vi "Init DB-Engine.vi"(6 "Database":string, 8 "error in":errorcluster, 9 "Password":string, 10 "User":string, 11 "DB-Engine in":refnum<class "DB-Interface.lvclass">) -> (0 "error out":errorcluster, 3 "DB-Engine out":refnum<class "DB-Interface.lvclass">)   [LabVIEW 2020, in "hse-db.lvlib" / "DB-Interface.lvclass"]
doc: "Initialize the class.\n\n____\nHAMPEL SOFTWARE ENGINEERING v1.4.0 (2023-12-19 09:52)"
uses:
  DB-Interface.lvclass
  DB-Interface.lvclass/DB-Interface.ctl
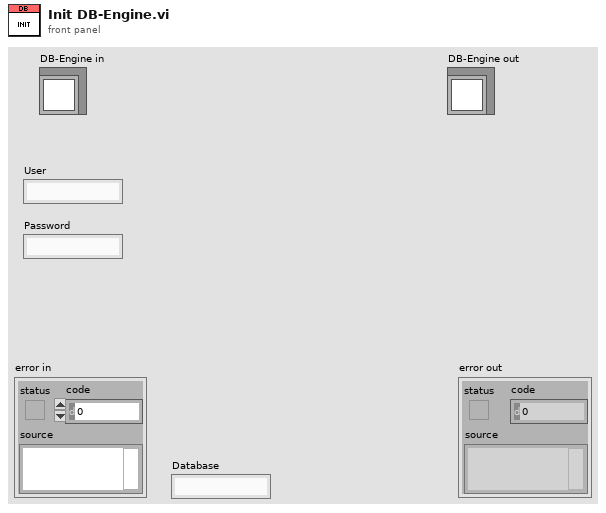
[diagram p1: front panel]
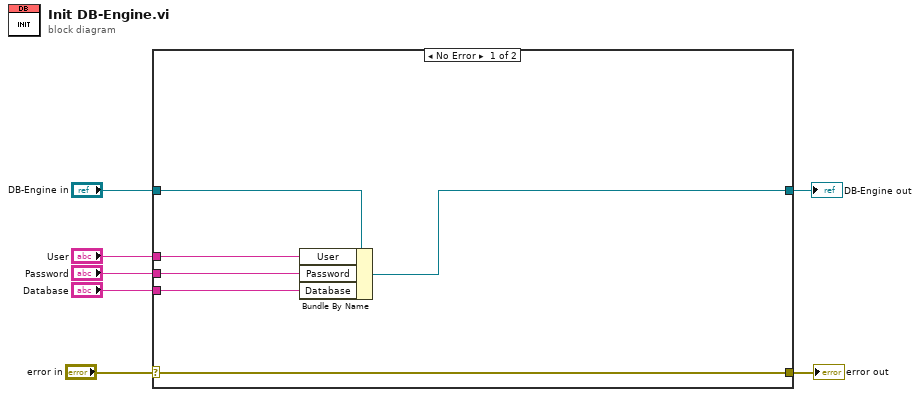
[diagram p0: block diagram]
diagram:
  n1 = case shown="No Error" "error in" {
    selector: "error in" -> [w13 w15]
    tunnel: [w13 w15] -> w6
    tunnel: [w12 w14] -> w5
    tunnel: "DB-Engine in" -> [w11 w14]
    tunnel: "User" -> [w10 _]
    tunnel: "Password" -> [w9 _]
    tunnel: "Database" -> [w8 _]
    frame No Error {
      n2 = Bundle By Name(cluster=w11, "User"=w10, "Password"=w9, "Database"=w8) -> (w12:refnum<class "DB-Interface.lvclass">)
    }
    frame Error {
    }
  }
  "error out" <- w6
  "DB-Engine out" <- w5
